vi "EXAMPLE - XML Config (Variant).vi"() -> ()   [LabVIEW 2013, in "XML Config.lvlib"]
uses:
  XML Config.lvlib
  <vilib>/vision/Image Controls.llb/IMAQ Image.ctl
panel:
  out "Settings":T1 {"Numeric" format="%#.11g"}
  in  "Settings":T1
  in  "Settings":T4={"Image path"=path "J:/Staple Images/Reference Staples 2014-09-29/Under/1 staple 2014-09-26T17.36.27 Composite Focus.tif", "Image Paths"=[], "Index"=0, "AutoContinue"=FALSE, "Image Type"=0, "Image In"=refnum, "Image Dst"=refnum, "Pre-Rotate"=0.0, "Angle, OverCrimp"=[], "Inspect Backplane"=TRUE, "Inspect OverCrimp"=TRUE, "Inspect UnderCrimp"=TRUE, "Upsample to"=0.0, "All Dir"=path "", "Folders"=[], "Folder Index"=0, "Angle, OuterLine"=[], "Angle, InnerLine"=[], "Angle, UnderCrimp"=[], "Cal Img Path"=path "C:/Projects/codedepot/Covidien/2014-1011 Covidien Automated Staple Measurement/Images/calibration/Calibration 2014-08-22T12.12.45/Calibration Template.png", "Numeric"=0.0} {"Numeric" format="%#.11g"; "Upsample to" min=0.0 max=4000.0 step=1.0; "Pre-Rotate" min=0.0 max=360.0 step=1.0; "Image Type" items=["Grayscale (U8)", "Grayscale (I16)", "Grayscale (SGL)", "Complex (CSG)", "RGB (U32)", "HSL (U32)", "RGB (U64)", "Grayscale (U16)"]}
  in  "Backplane Settings":T5={"Setup"={"Show Search Area"=FALSE, "Show Search Lines"=FALSE, "Show Edges Found"=FALSE, "Show Result"=TRUE}, "Outside Edge Options"={"Edge Polarity"=0, "Kernel Size"=13, "Width"=19, "Minimum Edge Strength"=100.0, "Interpolation Type"=enum."Zero Order", "Data Processing Method"=enum."Average"}, "Outside Line Options"={"Number of Lines"=1, "Type"=enum."First Edge Rake", "Min. Score"=0.0, "Max. Score"=1024.0, "Orientation"=0.0, "Angle Range"=40.0, "Angle Tolerance"=5.0, "Step Size"=20, "Min. SNR (db)"=0.0, "Min. Points (%)"=2.0, "Hough Iterations"=5}, "Settings Caliper"={"Contrast"=40, "Filter width"=4, "Steepness"=2, "Subsampling Ratio"=5, "Show Search Area"=FALSE, "Show Search Lines"=FALSE, "Show Edges Found"=FALSE, "Show Result"=FALSE}, "Look For (Bright Objects)"=1, "Method"=1, "Kernel Size"={"SizeX"=176, "SizeY"=176}, "Niblack Deviation Factor"=0.12, "Number of Erosion"=2, "Score Delineator"=150.0, "Auto Adjust Kernel Size"=TRUE, "Threshold Method"=0, "Use Quick method\nThreshold"=TRUE, "Scale Score"=TRUE, "Area Filter > 2"=10000.0, "Inside Edge Options"={"Edge Polarity"=2, "Kernel Size"=13, "Width"=19, "Minimum Edge Strength"=100.0, "Interpolation Type"=enum."Zero Order", "Data Processing Method"=enum."Average"}, "Inside Line Options"={"Number of Lines"=1, "Type"=enum."First Edge Rake", "Min. Score"=0.0, "Max. Score"=1024.0, "Orientation"=0.0, "Angle Range"=25.0, "Angle Tolerance"=1.0, "Step Size"=20, "Min. SNR (db)"=0.0, "Min. Points (%)"=1.0, "Hough Iterations"=5}, "Inner Width Reduce %"=30.0, "Inner Height Reduce %"=15.0, "Inner Setup"={"Show Search Area"=FALSE, "Show Search Lines"=FALSE, "Show Edges Found"=FALSE, "Show Result"=TRUE}, "Show CoM"=FALSE, "Keep All Results"=FALSE, "X Size"=0.0, "Y Size"=0.0} {"Inside Edge Options"."Edge Polarity" items=["All Edges", "Rising Edges", "Falling Edges"]; "Threshold Method" items=["clustering", "entropy", "metric", "moments", "inter-class variance"]; "Score Delineator" format="%#_15g"; "Niblack Deviation Factor" format="%#_15g"; "Method" items=["Niblack", "Background Correction"]; "Look For (Bright Objects)" items=["Bright Objects", "Dark Objects"]; "Outside Edge Options"."Edge Polarity" items=["All Edges", "Rising Edges", "Falling Edges"]}
  out "direct to variant":variant
  out "error out":errorcluster
  in  "Ring":u16(ring) items=["a", "b"]
  out "Variant out":variant
  in  "Cluster":T6={"Numeric"=0.0, "Boolean"=FALSE, "Template File Path"=path "C:/Projects/2010-4028/Vision Assistant Scripts/Wire Removal/Just U 7.png", "U Mask Offset"={"X"=5.0, "Y"=0.0}, "Array"=[]}
  out "XML":string="<Processing Settings>\n    <Number of Cameras>8</Number of Cameras>\r\n    <Image Dimensions>\n        <Total Chunks>7</Total Chunks>\r\n        <Lines per Chunk>1000</Lines per Chunk>\r\n    </Image Dimensions>\r\n    <Processing Settings>\n        <Process?>\n            <Broken Module>FALSE</Broken Module>\r\n            <Bubble - Vacuum>FALSE</Bubble - Vacuum>\r\n            <Bubble - Wire Closeness>FALSE</Bubble - Wire Closeness>\r\n            <Debris>FALSE</Debris>\r\n            <Edge Tape>FALSE</Edge Tape>\r\n            <Encapsulant to Glass Void>FALSE</Encapsulant to Glass Void>\r\n            <Glass Scratch>FALSE</Glass Scratch>\r\n            <J-Box to Glass Placement>FALSE</J-Box to Glass Placement>\r\n            <Potting Void - Exposed Lead>FALSE</Potting Void - Exposed Lead>\r\n            <Potting Void - Edge Zone Void>FALSE</Potting Void - Edge Zone Void>\r\n            <String Space>FALSE</String Space>\r\n            <Encapsulant Intrusion>FALSE</Encapsulant Intrusion>\r\n        </Process?>\r\n        <Edge Tape Parameters>\n            <Report Defects with Thickness Less Than (mm)>10</Report Defects with Thickness Less Than (mm)>\r\n            <Report Defects with Width Greater Than (mm)>0.5</Report Defects with Width Greater Than (mm)>\r\n            <Particle Filter Margin (mm)>3</Particle Filter Margin (mm)>\r\n            <Threshold Kernel Size>\n                <SizeX>429</SizeX>\r\n                <SizeY>429</SizeY>\r\n            </Threshold Kernel Size>\r\n            <Niblack Deviation Factor>0.2</Niblack Deviation Factor>\r\n            <Edge Options>\n                <Edge Polarity>0</Edge Polarity>\r\n                <Kernel Size>3</Kernel Size>\r\n                <Width>3</Width>\r\n                <Minimum Edge Strength>10</Minimum Edge Strength>\r\n                <Interpolation Type>4</Interpolation Type>\r\n                <Data Processing Method>0</Data Processing Method>\r\n            </Edge Options>\r\n            <Step Size (mm)>0.2</Step Size (mm)>\r\n            <Close Kernel Size (n x n)>0</Close Kernel Size (n x n)>\r\n            <Edge Tape Selection Margin (mm)>7</Edge Tape Selection Margin (mm)>\r\n            <Rake Inset Margin (mm)>5</Rake Inset Margin (mm)>\r\n            <Module Boundary Edge Options>\n                <Edge Polarity>0</Edge Polarity>\r\n                <Kernel Size>3</Kernel Size>\r\n                <Width>3</Width>\r\n                <Minimum Edge Strength>50</Minimum Edge Strength>\r\n                <Interpolation Type>4</Interpolation Type>\r\n                <Data Processing Method>0</Data Processing Method>\r\n            </Module Boundary Edge Options>\r\n            <Module Boundary Straight Edge Options>\n                <Number of Lines>1</Number of Lines>\r\n                <Type>0</Type>\r\n                <Min. Score>10</Min. Score>\r\n                <Max. Score>1000</Max. Score>\r\n                <Orientation>0</Orientation>\r\n                <Angle Range>45</Angle Range>\r\n                <Angle Tolerance>1</Angle Tolerance>\r\n                <Step Size>200</Step Size>\r\n                <Min. SNR (db)>0</Min. SNR (db)>\r\n                <Min. Points (%)>25</Min. Points (%)>\r\n                <Hough Iterations>5</Hough Iterations>\r\n            </Module Boundary Straight Edge Options>\r\n            <Number of Close Iterations>1</Number of Close Iterations>\r\n            <Edge Tape (Back) Threshold>\n                <Threshold Range, Percent of Full Range>25</Threshold Range, Percent of Full Range>\r\n                <Number of Classes>20</Number of Classes>\r\n                <Peak Detect Width>3</Peak Detect Width>\r\n                <Dismiss peaks >= N% of image area>35</Dismiss peaks >= N% of image area>\r\n                <Dismiss peaks <= N% of image area>0.2</Dismiss peaks <= N% of image area>\r\n                <Ideal Edge Tape Intensity (% of max)>30</Ideal Edge Tape Intensity (% of max)>\r\n                <Module Boundary Edge Options>\n                    <Edge Polarity>0</Edge Polarity>\r\n                    <Kernel Size>3</Kernel Size>\r\n                    <Width>3</Width>\r\n                    <Minimum Edge Strength>50</Minimum Edge Strength>\r\n                    <Interpolation Type>4</Interpolation Type>\r\n                    <Data Processing Method>0</Data Processing Method>\r\n                </Module Boundary Edge Options>\r\n                <Module Boundary Straight Edge Options>\n                    <Number of Lines>1</Number of Lines>\r\n                    <Type>0</Type>\r\n                    <Min. Score>10</Min. Score>\r\n                    <Max. Score>1000</Max. Score>\r\n                    <Orientation>0</Orientation>\r\n                    <Angle Range>45</Angle Range>\r\n                    <Angle Tolerance>1</Angle Tolerance>\r\n                    <Step Size>200</Step Size>\r\n                    <Min. SNR (db)>0</Min. SNR (db)>\r\n                    <Min. Points (%)>25</Min. Points (%)>\r\n                    <Hough Iterations>5</Hough Iterations>\r\n                </Module Boundary Straight Edge Options>\r\n                <J-Box Rake Inset Margin (mm)>5</J-Box Rake Inset Margin (mm)>\r\n                <Bottom Rake Inset Margin (mm)>5</Bottom Rake Inset Margin (mm)>\r\n            </Edge Tape (Back) Threshold>\r\n        </Edge Tape Parameters>\r\n        <J-Box Processing Parameters>\n            <Max J-Box Gap (mm)>0</Max J-Box Gap (mm)>\r\n        </J-Box Processing Parameters>\r\n        <String Space Cluster>\n            <Rough Find Threshold - %  Mean Increase>20</Rough Find Threshold - %  Mean Increase>\r\n            <Final Find Step Size>150</Final Find Step Size>\r\n            <Min Length (mm)>0</Min Length (mm)>\r\n            <Equalize?>FALSE</Equalize?>\r\n            <Edge Options>\n                <Edge Polarity>2</Edge Polarity>\r\n                <Kernel Size (Pixel)>11</Kernel Size (Pixel)>\r\n                <Width (Pixel)>3</Width (Pixel)>\r\n                <Minimum Edge Strength>78.849998</Minimum Edge Strength>\r\n                <Interpolation Type>0</Interpolation Type>\r\n                <Data Processing Method>0</Data Processing Method>\r\n            </Edge Options>\r\n            <Max Length (mm)>0</Max Length (mm)>\r\n            <Grey Morphology?>FALSE</Grey Morphology?>\r\n        </String Space Cluster>\r\n        <Wire Removal - U Find Cluster>\n            <U Pattern Match Find Cluster>\n                <Minimum Match Score>700</Minimum Match Score>\r\n                <Template U Pattern Match Array>\n                </Template U Pattern Match Array>\r\n            </U Pattern Match Find Cluster>\r\n            <U Pattern Match to Wire Mask ROI Cluster>\n                <Group U Points By Cell Cluster>\n                    <# Bins>200</# Bins>\r\n                    <Wire Seperation Threshold (%)>10</Wire Seperation Threshold (%)>\r\n                    <Min # Points>5</Min # Points>\r\n                </Group U Points By Cell Cluster>\r\n                <Dead Reckon - Y Spacing Threshold (%)>45</Dead Reckon - Y Spacing Threshold (%)>\r\n                <Wire ROI Descriptive Cluster>\n                    <ROI Open Direction></ROI Open Direction>\r\n                    <Wire ROI Dimensions>\n                        <L>20</L>\r\n                        <H>44</H>\r\n                        <Wh>14</Wh>\r\n                        <Wv>10</Wv>\r\n                    </Wire ROI Dimensions>\r\n                </Wire ROI Descriptive Cluster>\r\n                <Duplicate Removal Seperation Threshold (%)>45</Duplicate Removal Seperation Threshold (%)>\r\n            </U Pattern Match to Wire Mask ROI Cluster>\r\n            <Cell Edge Detect and Mask Create Cluster>\n                <Search Direction>0</Search Direction>\r\n                <Line Options>\n                    <Number of Lines>1</Number of Lines>\r\n                    <Type>4</Type>\r\n                    <Min. Score>0</Min. Score>\r\n                    <Max. Score>1024</Max. Score>\r\n                    <Orientation>0</Orientation>\r\n                    <Angle Range>20</Angle Range>\r\n                    <Angle Tolerance>0.01</Angle Tolerance>\r\n                    <Step Size>3</Step Size>\r\n                    <Min. SNR (db)>0</Min. SNR (db)>\r\n                    <Min. Points (%)>25</Min. Points (%)>\r\n                    <Hough Iterations>5</Hough Iterations>\r\n                </Line Options>\r\n                <Edge Options>\n                    <Edge Polarity>1</Edge Polarity>\r\n                    <Kernel Size>15</Kernel Size>\r\n                    <Width>3</Width>\r\n                    <Minimum Edge Strength>24.705883</Minimum Edge Strength>\r\n                    <Interpolation Type>0</Interpolation Type>\r\n                    <Data Processing Method>0</Data Processing Method>\r\n                </Edge Options>\r\n                <Cell Search ROI Width>100</Cell Search ROI Width>\r\n                <Cell Mask ROI Width>25</Cell Mask ROI Width>\r\n            </Cell Edge Detect and Mask Create Cluster>\r\n        </Wire Removal - U Find Cluster>\r\n        <Wire Parameters Cluster>\n            <Wire Lenght (mm)>28.299999</Wire Lenght (mm)>\r\n            <Wire Vertical Seperation Distance (mm)>5.7</Wire Vertical Seperation Distance (mm)>\r\n        </Wire Parameters Cluster>\r\n        <Broken Module Settings>\n            <Morphology>\n                <Iterations>3</Iterations>\r\n                <Operation>1</Operation>\r\n                <Stucturing Element>\n                    <element 0:0>\n                                        <Numeric>1</Numeric>\n                    </element 0:0>\r\n                    <element 1:0>\n                                        <Numeric>1</Numeric>\n                    </element 1:0>\r\n                    <element 2:0>\n                                        <Numeric>1</Numeric>\n                    </element 2:0>\r\n                    <element 3:0>\n                                        <Numeric>1</Numeric>\n                    </element 3:0>\r\n                    <element 4:0>\n                                        <Numeric>1</Numeric>\n                    </element 4:0>\r\n                    <element 0:1>\n                                        <Numeric>1</Numeric>\n                    </element 0:1>\r\n                    <element 1:1>\n                                        <Numeric>1</Numeric>\n                    </element 1:1>\r\n                    <element 2:1>\n                                        <Numeric>1</Numeric>\n                    </element 2:1>\r\n                    <element 3:1>\n                                        <Numeric>1</Numeric>\n                    </element 3:1>\r\n                    <element 4:1>\n                                        <Numeric>1</Numeric>\n                    </element 4:1>\r\n                    <element 0:2>\n                                        <Numeric>1</Numeric>\n                    </element 0:2>\r\n                    <element 1:2>\n                                        <Numeric>1</Numeric>\n                    </element 1:2>\r\n                    <element 2:2>\n                                        <Numeric>1</Numeric>\n                    </element 2:2>\r\n                    <element 3:2>\n                                        <Numeric>1</Numeric>\n                    </element 3:2>\r\n                    <element 4:2>\n                                        <Numeric>1</Numeric>\n                    </element 4:2>\r\n                    <element 0:3>\n                                        <Numeric>1</Numeric>\n                    </element 0:3>\r\n                    <element 1:3>\n                                        <Numeric>1</Numeric>\n                    </element 1:3>\r\n                    <element 2:3>\n                                        <Numeric>1</Numeric>\n                    </element 2:3>\r\n                    <element 3:3>\n                                        <Numeric>1</Numeric>\n                    </element 3:3>\r\n                    <element 4:3>\n                                        <Numeric>1</Numeric>\n                    </element 4:3>\r\n                    <element 0:4>\n                                        <Numeric>1</Numeric>\n                    </element 0:4>\r\n                    <element 1:4>\n                                        <Numeric>1</Numeric>\n                    </element 1:4>\r\n                    <element 2:4>\n                                        <Numeric>1</Numeric>\n                    </element 2:4>\r\n                    <element 3:4>\n                                        <Numeric>1</Numeric>\n                    </element 3:4>\r\n                    <element 4:4>\n                                        <Numeric>1</Numeric>\n                    </element 4:4>\r\n                </Stucturing Element>\r\n            </Morphology>\r\n            <NI Black Settings>\n                <Method>1</Method>\r\n                <Look For>1</Look For>\r\n                <Kernel Size>\n                    <SizeY>75</SizeY>\r\n                    <SizeX>75</SizeX>\r\n                </Kernel Size>\r\n                <Deviation Factor>0.2</Deviation Factor>\r\n            </NI Black Settings>\r\n            <Check Standard Variation Failure >>0.35</Check Standard Variation Failure >>\r\n        </Broken Module Settings>\r\n    </Processing Settings>\r\n    <Camera Scale Factor Array>\n        <element 0>\n                <Camera Scale Factor>\n            <Module Side></Module Side>\r\n            <Camera></Camera>\r\n            <Pixels / mm>\n                <X>10</X>\r\n                <Y>10</Y>\r\n            </Pixels / mm>\r\n            <Quality Score>0</Quality Score>\r\n        </Camera Scale Factor>\n        </element 0>\r\n        <element 1>\n                <Camera Scale Factor>\n            <Module Side></Module Side>\r\n            <Camera></Camera>\r\n            <Pixels / mm>\n                <X>10</X>\r\n                <Y>10</Y>\r\n            </Pixels / mm>\r\n            <Quality Score>0</Quality Score>\r\n        </Camera Scale Factor>\n        </element 1>\r\n        <element 2>\n                <Camera Scale Factor>\n            <Module Side></Module Side>\r\n            <Camera></Camera>\r\n            <Pixels / mm>\n                <X>10</X>\r\n                <Y>10</Y>\r\n            </Pixels / mm>\r\n            <Quality Score>0</Quality Score>\r\n        </Camera Scale Factor>\n        </element 2>\r\n        <element 3>\n                <Camera Scale Factor>\n            <Module Side></Module Side>\r\n            <Camera></Camera>\r\n            <Pixels / mm>\n                <X>10</X>\r\n                <Y>10</Y>\r\n            </Pixels / mm>\r\n            <Quality Score>0</Quality Score>\r\n        </Camera Scale Factor>\n        </element 3>\r\n        <element 4>\n                <Camera Scale Factor>\n            <Module Side></Module Side>\r\n            <Camera></Camera>\r\n            <Pixels / mm>\n                <X>10</X>\r\n                <Y>10</Y>\r\n            </Pixels / mm>\r\n            <Quality Score>0</Quality Score>\r\n        </Camera Scale Factor>\n        </element 4>\r\n        <element 5>\n                <Camera Scale Factor>\n            <Module Side></Module Side>\r\n            <Camera></Camera>\r\n            <Pixels / mm>\n                <X>10</X>\r\n                <Y>10</Y>\r\n            </Pixels / mm>\r\n            <Quality Score>0</Quality Score>\r\n        </Camera Scale Factor>\n        </element 5>\r\n        <element 6>\n                <Camera Scale Factor>\n            <Module Side></Module Side>\r\n            <Camera></Camera>\r\n            <Pixels / mm>\n                <X>10</X>\r\n                <Y>10</Y>\r\n            </Pixels / mm>\r\n            <Quality Score>0</Quality Score>\r\n        </Camera Scale Factor>\n        </element 6>\r\n        <element 7>\n                <Camera Scale Factor>\n            <Module Side></Module Side>\r\n            <Camera></Camera>\r\n            <Pixels / mm>\n                <X>10</X>\r\n                <Y>10</Y>\r\n            </Pixels / mm>\r\n            <Quality Score>0</Quality Score>\r\n        </Camera Scale Factor>\n        </element 7>\r\n    </Camera Scale Factor Array>\r\n</Processing Settings>"
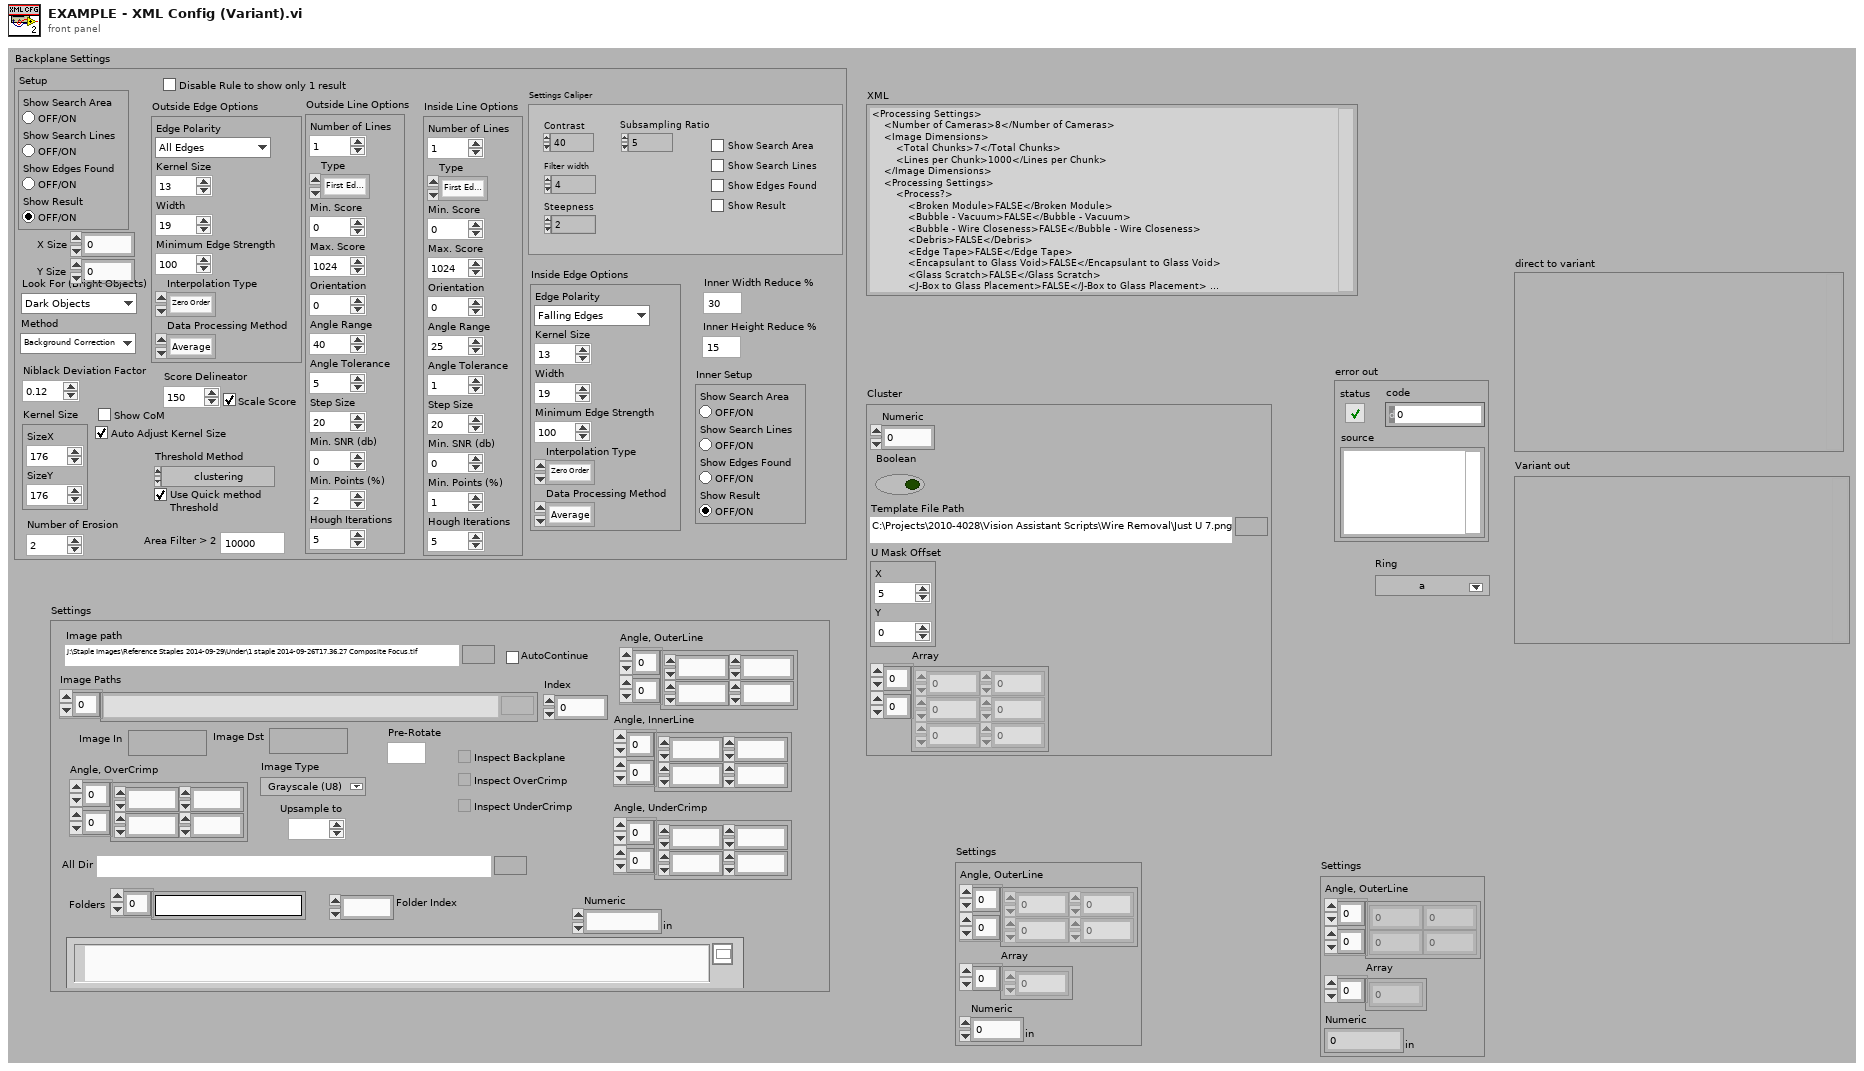
[diagram p1: front panel]
types:
  T1 = cluster{"Angle, OuterLine":dbl[][], "Array":dbl[], "Numeric":dbl[unit]}
  T2 = typedef "Image Type" = u32
  T3 = typedef "IMAQ Image.ctl" = refnum<image>
  T4 = cluster{"Image path":path, "Image Paths":path[], "Index":u32, "AutoContinue":bool, "Image Type":T2, "Image In":T3, "Image Dst":T3, "Pre-Rotate":dbl, "Angle, OverCrimp":dbl[][], "Inspect Backplane":bool, "Inspect OverCrimp":bool, "Inspect UnderCrimp":bool, "Upsample to":dbl, "All Dir":path, "Folders":string[], "Folder Index":u32, "Angle, OuterLine":dbl[][], "Angle, InnerLine":dbl[][], "Angle, UnderCrimp":dbl[][], "Cal Img Path":path, "Numeric":dbl[unit]}
  T5 = cluster{"Setup":cluster{"Show Search Area":bool, "Show Search Lines":bool, "Show Edges Found":bool, "Show Result":bool}, "Outside Edge Options":cluster{"Edge Polarity":u32, "Kernel Size":u32, "Width":u32, "Minimum Edge Strength":sgl, "Interpolation Type":enum32{"Zero Order", "Bilinear", "Quadratic", "Cubic", "Bilinear Fixed"}, "Data Processing Method":enum32{"Average", "Median"}}, "Outside Line Options":cluster{"Number of Lines":i32, "Type":enum32{"First Edge Rake", "Best Edge Rake", "Hough Edge Rake", "First Edge Projection", "Best Edge Projection"}, "Min. Score":dbl, "Max. Score":dbl, "Orientation":dbl, "Angle Range":dbl, "Angle Tolerance":dbl, "Step Size":u32, "Min. SNR (db)":dbl, "Min. Points (%)":dbl, "Hough Iterations":i32}, "Settings Caliper":cluster{"Contrast":i32, "Filter width":i32, "Steepness":i32, "Subsampling Ratio":u32, "Show Search Area":bool, "Show Search Lines":bool, "Show Edges Found":bool, "Show Result":bool}, "Look For (Bright Objects)":u32, "Method":u32, "Kernel Size":cluster{"SizeX":i32, "SizeY":i32}, "Niblack Deviation Factor":dbl, "Number of Erosion":i32, "Score Delineator":dbl, "Auto Adjust Kernel Size":bool, "Threshold Method":i32, "Use Quick method\nThreshold":bool, "Scale Score":bool, "Area Filter > 2":dbl, "Inside Edge Options":cluster{"Edge Polarity":u32, "Kernel Size":u32, "Width":u32, "Minimum Edge Strength":sgl, "Interpolation Type":enum32{"Zero Order", "Bilinear", "Quadratic", "Cubic", "Bilinear Fixed"}, "Data Processing Method":enum32{"Average", "Median"}}, "Inside Line Options":cluster{"Number of Lines":i32, "Type":enum32{"First Edge Rake", "Best Edge Rake", "Hough Edge Rake", "First Edge Projection", "Best Edge Projection"}, "Min. Score":dbl, "Max. Score":dbl, "Orientation":dbl, "Angle Range":dbl, "Angle Tolerance":dbl, "Step Size":u32, "Min. SNR (db)":dbl, "Min. Points (%)":dbl, "Hough Iterations":i32}, "Inner Width Reduce %":dbl, "Inner Height Reduce %":dbl, "Inner Setup":cluster{"Show Search Area":bool, "Show Search Lines":bool, "Show Edges Found":bool, "Show Result":bool}, "Show CoM":bool, "Keep All Results":bool, "X Size":dbl, "Y Size":dbl}
  T6 = cluster{"Numeric":dbl, "Boolean":bool, "Template File Path":path, "U Mask Offset":cluster{"X":sgl, "Y":sgl}, "Array":dbl[][]}
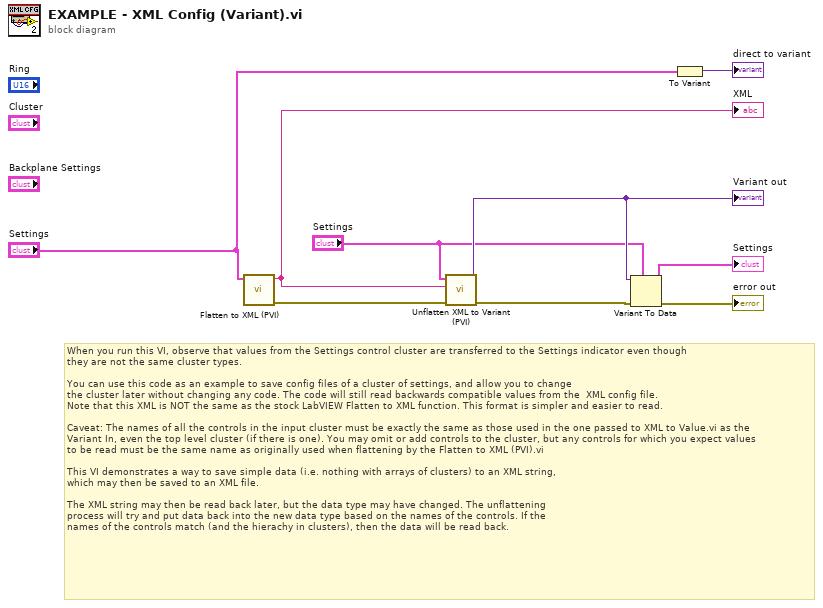
[diagram p0: block diagram]
diagram:
  # "When you run this VI, observe that values from the Settings control cluster are transferred to the Settings indicator even though\nthey are not the same cluster types.\n\nYou can use this code as an example to save config files of a cluster of settings, and allow you to change\nthe cluster later without changing any code. The code will still read backwards compatible values from the  XML config file.\nNote that this XML is NOT the same as the stock LabVIEW Flatten to XML function. This format is simpler and easier to read.\n\nCaveat: The names of all the controls in the input cluster must be exactly the same as those used in the one passed to XML to Value.vi as the\nVariant In, even the top level cluster (if there is one). You may omit or add controls to the cluster, but any controls for which you expect values\nto be read must be the same name as originally used when flattening by the Flatten to XML (PVI).vi\n\nThis VI demonstrates a way to save simple data (i.e. nothing with arrays of clusters) to an XML string,\nwhich may then be saved to an XML file.\n\nThe XML string may then be read back later, but the data type may have changed. The unflattening\nprocess will try and put data back into the new data type based on the names of the controls. If the\nnames of the controls match (and the hierachy in clusters), then the data will be read back."
  n1 = call "Flatten to XML (PVI).vi"("Variant"="Settings") -> ("error out"=w1:errorcluster, "XML"=w6:string)  [unwired: 9 in]
  "XML" <- w6
  n2 = call "Unflatten XML to Variant (PVI).vi"("error in (no error)"=w1, "XML"=w6, "Variant in (for type and default data)"="Settings") -> ("error out"=w5:errorcluster, "Variant out"=w9:variant)  [unwired: 7 in]
  "Variant out" <- w9
  n3 = Variant To Data(error in=w5, type="Settings", Variant=w9) -> (data=→"Settings":T1, error out=→"error out":errorcluster)
  n4 = To Variant(anything="Settings") -> (Variant=→"direct to variant":variant)
